vi "Get System Tag Path.vi"(11 "sytem tag":T1) -> (3 "tag path":string)   [LabVIEW 2020, in "FlexLoggerTagHelpers.lvlib"]
uses:
  FlexLoggerTagHelpers.lvlib
  System Tags.ctl
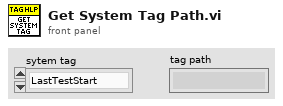
[diagram p1: front panel]
types:
  T1 = typedef "FlexLoggerTagHelpers.lvlib/System Tags.ctl" = enum16{"LastTestStart", "IsTestSessionRunning"}
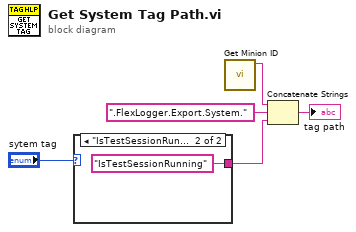
[diagram p0: block diagram]
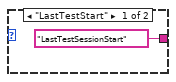
[diagram p2: hidden frame]
diagram:
  n1 = case shown="\"IsTestSessionRunning\"" "sytem tag" {
    tunnel: ["LastTestSessionStart" ("string") "IsTestSessionRunning" ("string")] -> w1
    frame "LastTestStart" {
    }
    frame "IsTestSessionRunning" {
    }
  }
  n2 = call <vilib>:"Get Minion ID.vi"() -> ("minion id"=w4:string)  [unwired: 11 in]
  n3 = Concatenate Strings(w4, ".FlexLogger.Export.System." ("string"), w1) -> (→"tag path":string)
